vi "Overview.vi"() -> ()   [LabVIEW 2017]
panel:
  out "CTAH Temp In Res":dbl(graph)
  out "Heater Temp Out Res":dbl(graph)
  out "TCHX Temp In Res":dbl(graph)
  out "DHX Temp Out Res":dbl(graph)
  out "CTAH Heat Removal Res":dbl(graph)
  out "Heater Control Res":dbl(graph)
  out "Natural Gas Flow [kg/s]":sgl caption="C" format="%_3f"
  out "Time [s]":sgl format="%.1f"
  out "Primary Flow [kg/s]":sgl caption="C" format="%_3f"
  out "TCHX Power [W]":sgl caption="C" format="%_3f"
  out "DHX Power [W]":sgl caption="C" format="%_3f"
  out "Electrical Power [W]":sgl format="%_3f"
  in  "stop":bool
  out "Primary Min Temp [C]":sgl format="%_3f"
  out "CTAH Power [W]":sgl format="%_3f"
  out "Primary Max Temp [C]":sgl format="%_3f"
  out "Heater Power [W]":sgl caption="C" format="%_3f"
  out "LPT Work [W]":sgl format="%_3f"
  out "HPT Work [W]":sgl format="%_3f"
  out "Compressor Work [W]":sgl format="%_3f"
  out "Ambient Temperature [C]":sgl format="%_3f"
  # "Overview"
  # "TCHX"
  # "LPT"
  # "HPT"
  # "COMPRESSOR"
  # "DHX"
  # "CTAH"
  # "COMBUSTOR"
  # "HEATER"
  # "PUMP"
  # "NOAH Jr."
  # "Procedures"
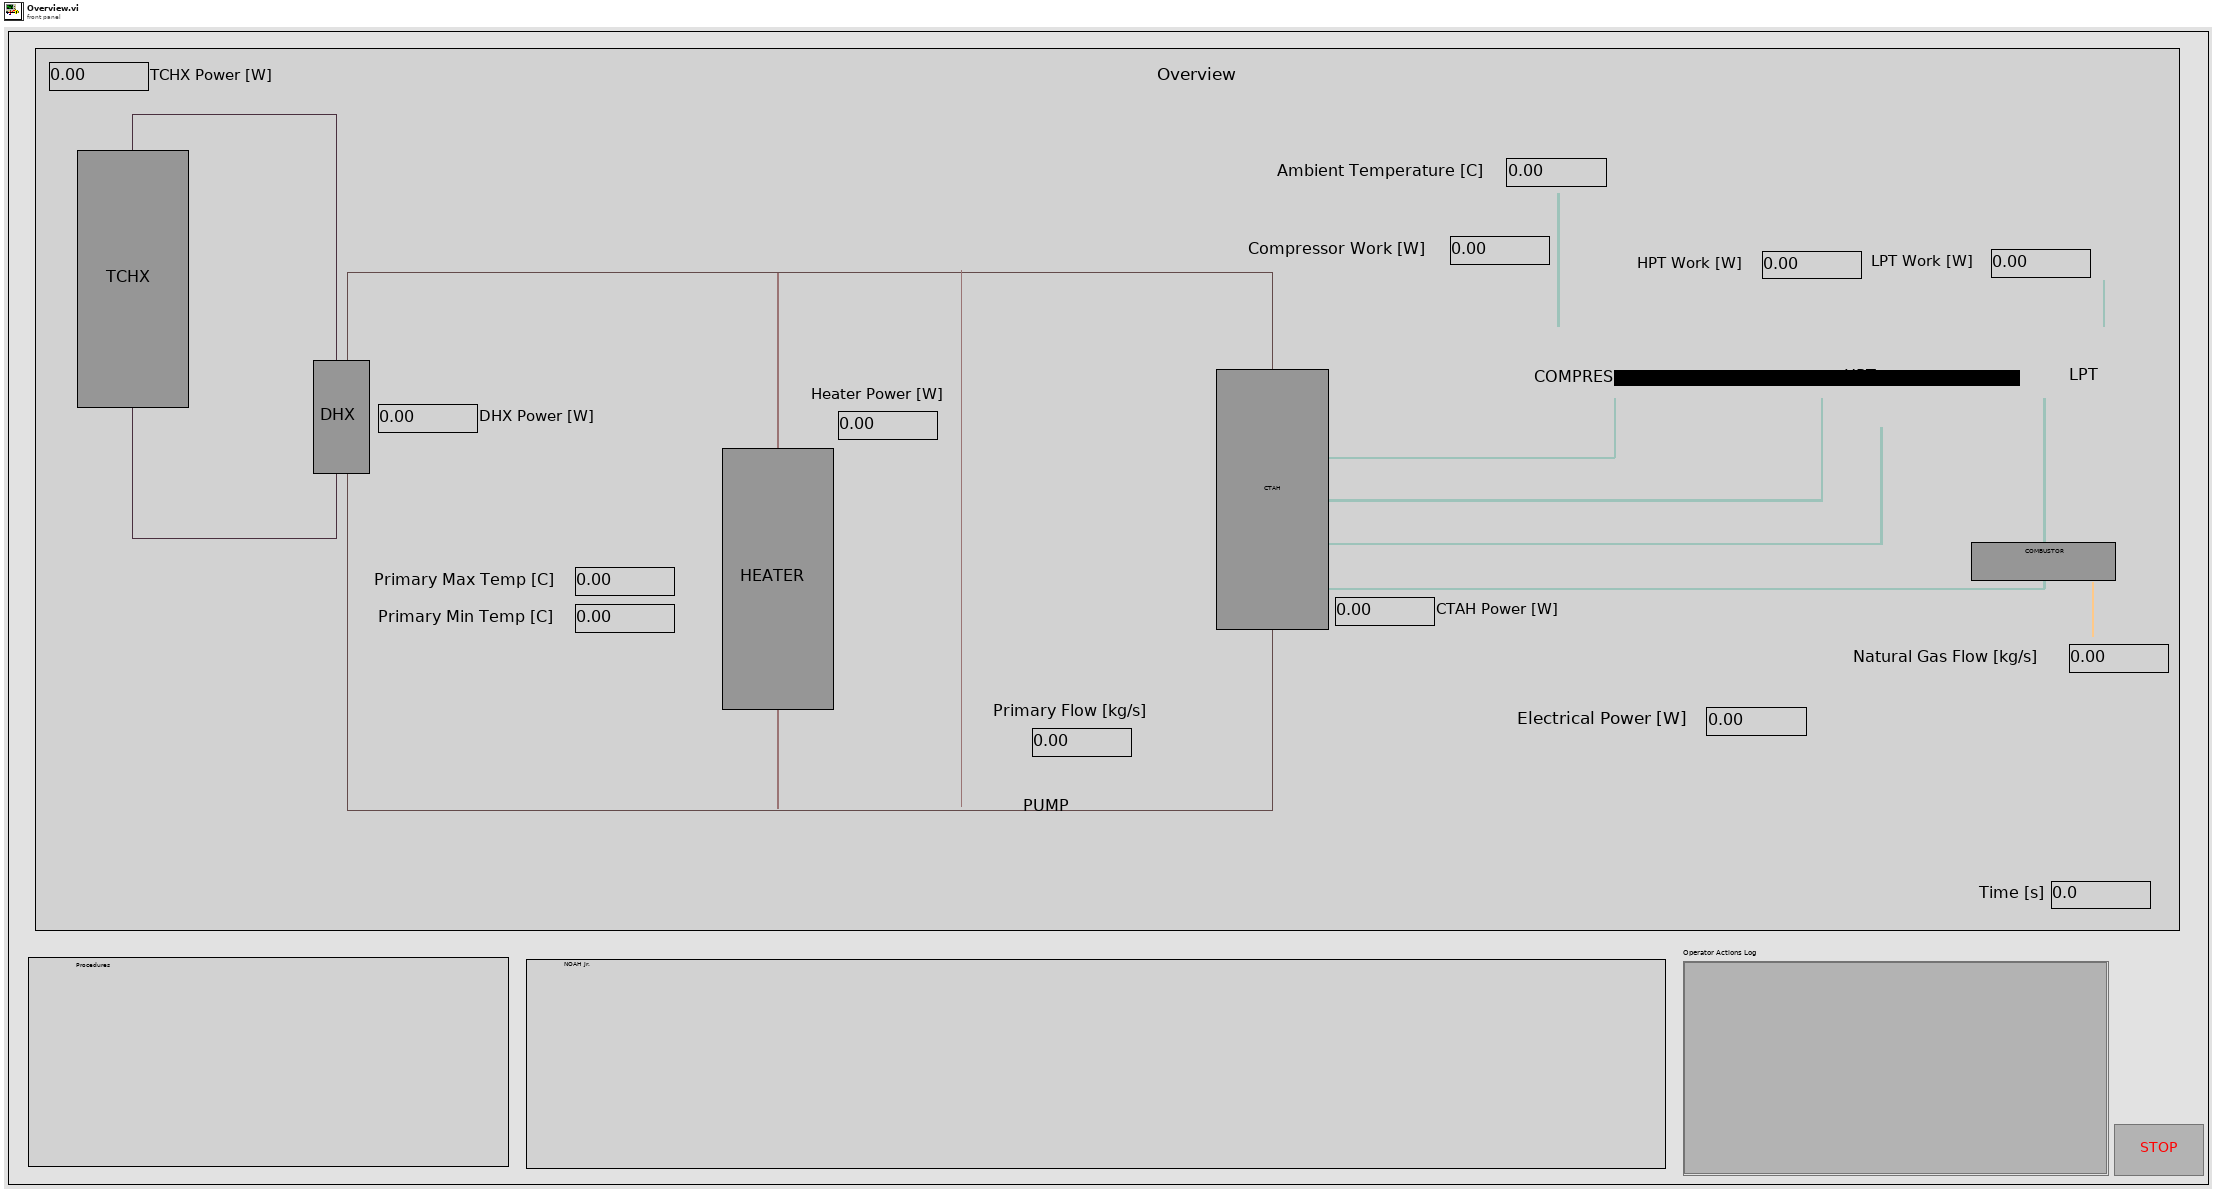
[diagram p1: front panel]
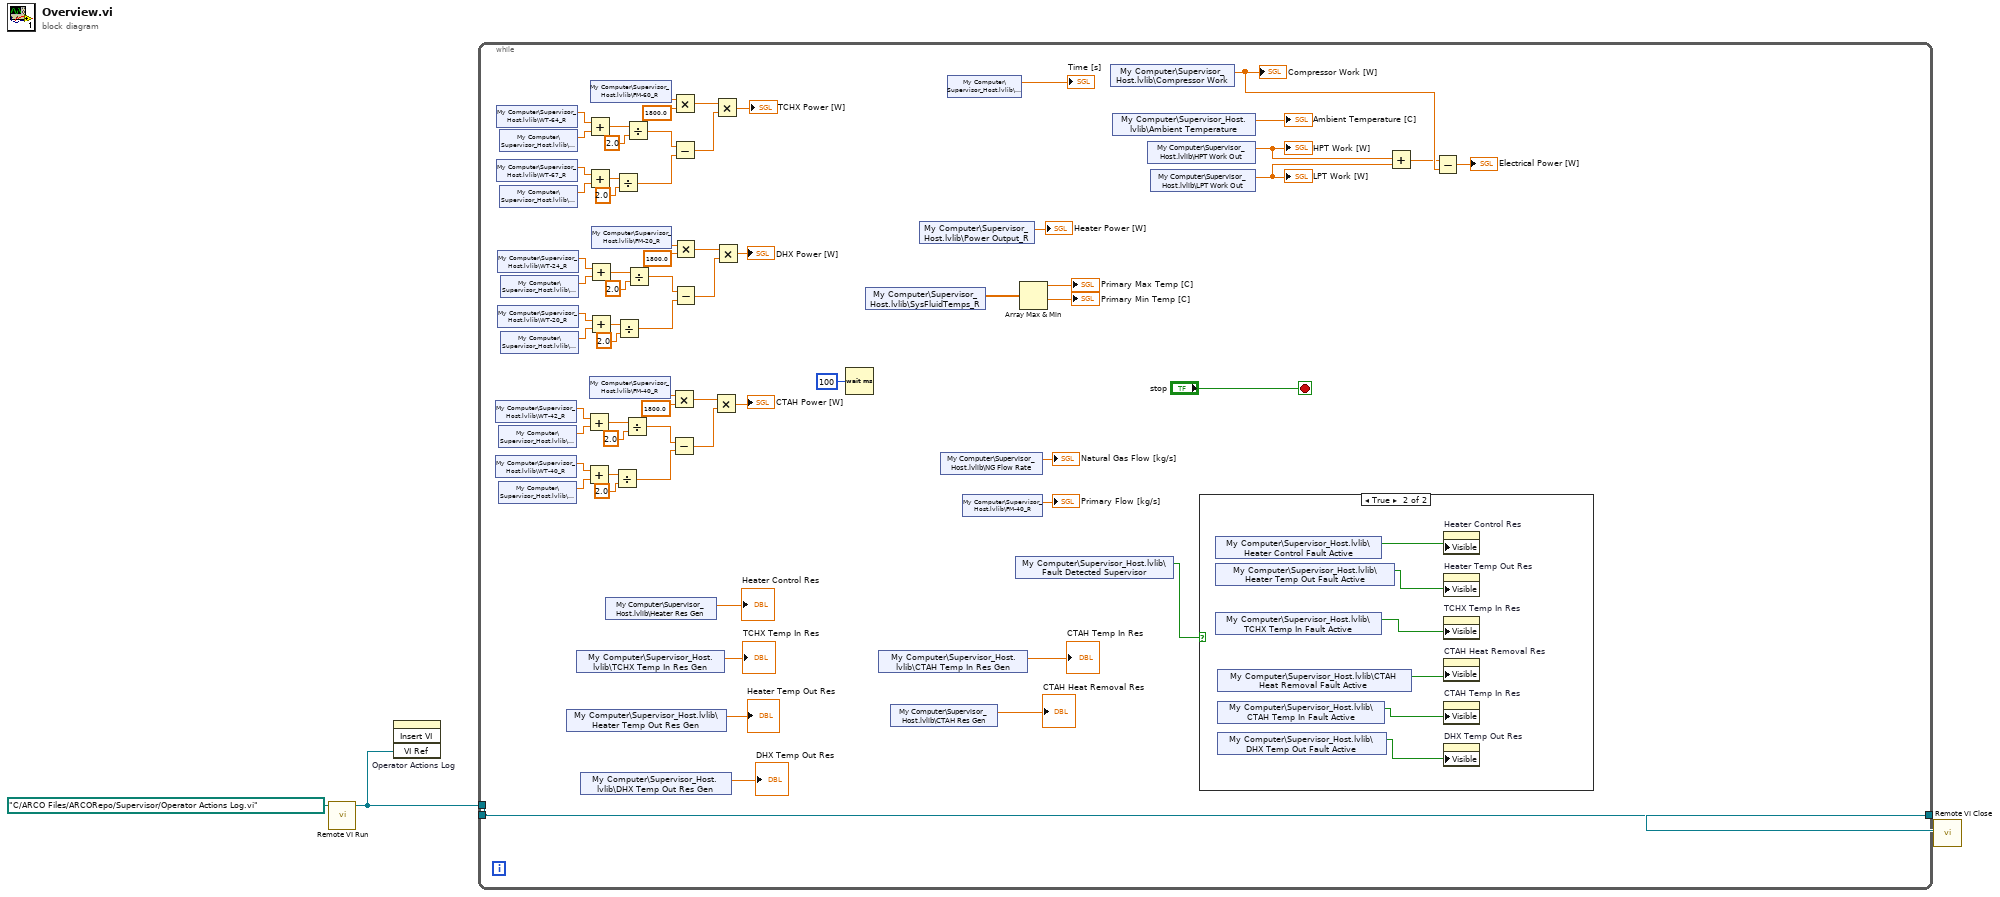
[diagram p0: block diagram]
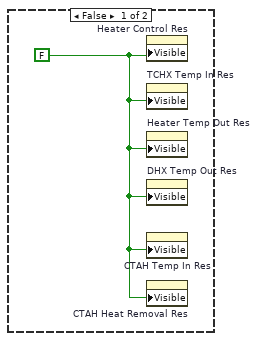
[diagram p2: hidden frame]
diagram:
  n1 = call "Remote VI Run.vi"("VI Path"=path "C:/ARCO Files/ARCORepo/Supervisor/Operator Actions Log.vi") -> ("VI Reference"=w2:refnum<vi>)  [unwired: 9 in, 1 out]
  n2 = invoke on="Operator Actions Log" class="SubPnl" method="Insert VI"("VI Ref"=w2) -> ()  [unwired: 3 in, 4 out]
  n3 = while {
    tunnel: [w5] -> _
    tunnel: w2 -> [w5]
    tunnel: [w5] -> w1
    stop <- "stop" stop-if-true
    n4 = shared-variable "My Computer\\Supervisor_Host.lvlib\\WT-42_R"() -> (w26:sgl)  [unwired: 1 in, 1 out]
    n5 = shared-variable "My Computer\\Supervisor_Host.lvlib\\WT-40_R"() -> (w23:sgl)  [unwired: 1 in, 1 out]
    n6 = shared-variable "My Computer\\Supervisor_Host.lvlib\\WT-64_R"() -> (w54:sgl)  [unwired: 1 in, 1 out]
    n7 = shared-variable "My Computer\\Supervisor_Host.lvlib\\WT-67_R"() -> (w51:sgl)  [unwired: 1 in, 1 out]
    n8 = shared-variable "My Computer\\Supervisor_Host.lvlib\\WT-24_R"() -> (w40:sgl)  [unwired: 1 in, 1 out]
    n9 = shared-variable "My Computer\\Supervisor_Host.lvlib\\WT-20_R"() -> (w37:sgl)  [unwired: 1 in, 1 out]
    n10 = shared-variable "My Computer\\Supervisor_Host.lvlib\\BT-43_R"() -> (w27:sgl)  [unwired: 1 in, 1 out]
    n11 = shared-variable "My Computer\\Supervisor_Host.lvlib\\BT-41_R"() -> (w22:sgl)  [unwired: 1 in, 1 out]
    n12 = shared-variable "My Computer\\Supervisor_Host.lvlib\\BT-65_R"() -> (w55:sgl)  [unwired: 1 in, 1 out]
    n13 = shared-variable "My Computer\\Supervisor_Host.lvlib\\BT-66_R"() -> (w50:sgl)  [unwired: 1 in, 1 out]
    n14 = shared-variable "My Computer\\Supervisor_Host.lvlib\\BT-25_R"() -> (w41:sgl)  [unwired: 1 in, 1 out]
    n15 = shared-variable "My Computer\\Supervisor_Host.lvlib\\BT-21_R"() -> (w36:sgl)  [unwired: 1 in, 1 out]
    n16 = shared-variable "My Computer\\Supervisor_Host.lvlib\\Heater Temp Out Res Gen"() -> (→"Heater Temp Out Res":dbl)  [unwired: 1 in, 1 out]
    n17 = shared-variable "My Computer\\Supervisor_Host.lvlib\\TCHX Temp In Res Gen"() -> (→"TCHX Temp In Res":dbl)  [unwired: 1 in, 1 out]
    n18 = shared-variable "My Computer\\Supervisor_Host.lvlib\\DHX Temp Out Res Gen"() -> (→"DHX Temp Out Res":dbl)  [unwired: 1 in, 1 out]
    n19 = Add(x=w26, y=w27) -> (x+y=w25:sgl)
    n20 = Add(x=w23, y=w22) -> (x+y=w21:sgl)
    n21 = Add(x=w54, y=w55) -> (x+y=w53:sgl)
    n22 = Add(x=w51, y=w50) -> (x+y=w49:sgl)
    n23 = Add(x=w40, y=w41) -> (x+y=w39:sgl)
    n24 = Add(x=w37, y=w36) -> (x+y=w35:sgl)
    n25 = shared-variable "My Computer\\Supervisor_Host.lvlib\\FM-40_R"() -> (w29:sgl)  [unwired: 1 in, 1 out]
    n26 = shared-variable "My Computer\\Supervisor_Host.lvlib\\FM-60_R"() -> (w57:sgl)  [unwired: 1 in, 1 out]
    n27 = shared-variable "My Computer\\Supervisor_Host.lvlib\\FM-20_R"() -> (w43:sgl)  [unwired: 1 in, 1 out]
    n28 = shared-variable "My Computer\\Supervisor_Host.lvlib\\Heater Res Gen"() -> (→"Heater Control Res":dbl)  [unwired: 1 in, 1 out]
    n29 = Divide(x=w21, y=sgl 2.0) -> (x/y=w18:sgl)
    n30 = Divide(x=w49, y=sgl 2.0) -> (x/y=w46:sgl)
    n31 = Divide(x=w35, y=sgl 2.0) -> (x/y=w32:sgl)
    n32 = Divide(x=w25, y=sgl 2.0) -> (x/y=w19:sgl)
    n33 = Divide(x=w53, y=sgl 2.0) -> (x/y=w47:sgl)
    n34 = Divide(x=w39, y=sgl 2.0) -> (x/y=w33:sgl)
    n35 = Multiply(x=w29, y=sgl 1800.0) -> (x*y=w17:sgl)
    n36 = Subtract(x=w19, y=w18) -> (x-y=w16:sgl)
    n37 = Multiply(x=w57, y=sgl 1800.0) -> (x*y=w45:sgl)
    n38 = Subtract(x=w47, y=w46) -> (x-y=w44:sgl)
    n39 = Multiply(x=w43, y=sgl 1800.0) -> (x*y=w31:sgl)
    n40 = Subtract(x=w33, y=w32) -> (x-y=w30:sgl)
    n41 = Multiply(x=w17, y=w16) -> (x*y=→"CTAH Power [W]":sgl)
    n42 = Multiply(x=w45, y=w44) -> (x*y=→"TCHX Power [W]":sgl)
    n43 = Multiply(x=w31, y=w30) -> (x*y=→"DHX Power [W]":sgl)
    n44 = Wait (ms)(milliseconds to wait=u32 100) -> ()  [unwired: 1 out]
    n45 = shared-variable "My Computer\\Supervisor_Host.lvlib\\SysFluidTemps_R"() -> (w70:sgl[])  [unwired: 1 in, 1 out]
    n46 = shared-variable "My Computer\\Supervisor_Host.lvlib\\CTAH Temp In Res Gen"() -> (→"CTAH Temp In Res":dbl)  [unwired: 1 in, 1 out]
    n47 = shared-variable "My Computer\\Supervisor_Host.lvlib\\CTAH Res Gen"() -> (→"CTAH Heat Removal Res":dbl)  [unwired: 1 in, 1 out]
    n48 = shared-variable "My Computer\\Supervisor_Host.lvlib\\Power Output_R"() -> (→"Heater Power [W]":sgl)  [unwired: 1 in, 1 out]
    n49 = shared-variable "My Computer\\Supervisor_Host.lvlib\\NG Flow Rate"() -> (→"Natural Gas Flow [kg/s]":sgl)  [unwired: 1 in, 1 out]
    n50 = shared-variable "My Computer\\Supervisor_Host.lvlib\\Time_R"() -> (→"Time [s]":sgl)  [unwired: 1 in, 1 out]
    n51 = shared-variable "My Computer\\Supervisor_Host.lvlib\\FM-40_R"() -> (→"Primary Flow [kg/s]":sgl)  [unwired: 1 in, 1 out]
    n52 = shared-variable "My Computer\\Supervisor_Host.lvlib\\Fault Detected Supervisor"() -> (w4:bool)  [unwired: 1 in, 1 out]
    n53 = Array Max & Min(array=w70) -> (max value=→"Primary Max Temp [C]":sgl, min value=→"Primary Min Temp [C]":sgl)  [unwired: 2 out]
    n54 = shared-variable "My Computer\\Supervisor_Host.lvlib\\Compressor Work"() -> (w61:sgl)  [unwired: 1 in, 1 out]
    "Compressor Work [W]" <- w61
    n55 = shared-variable "My Computer\\Supervisor_Host.lvlib\\Ambient Temperature"() -> (→"Ambient Temperature [C]":sgl)  [unwired: 1 in, 1 out]
    n56 = shared-variable "My Computer\\Supervisor_Host.lvlib\\HPT Work Out"() -> (w63:sgl)  [unwired: 1 in, 1 out]
    "HPT Work [W]" <- w63
    n57 = shared-variable "My Computer\\Supervisor_Host.lvlib\\LPT Work Out"() -> (w62:sgl)  [unwired: 1 in, 1 out]
    "LPT Work [W]" <- w62
    n58 = case shown="True" w4 {
      frame False {
        w72 = FALSE
        n59 = property on="Heater Control Res" class="WFChart (strict)"("Visible"=w72) -> ()  [unwired: 2 in, 2 out]
        n60 = property on="TCHX Temp In Res" class="WFChart (strict)"("Visible"=w72) -> ()  [unwired: 2 in, 2 out]
        n61 = property on="Heater Temp Out Res" class="WFChart (strict)"("Visible"=w72) -> ()  [unwired: 2 in, 2 out]
        n62 = property on="DHX Temp Out Res" class="WFChart (strict)"("Visible"=w72) -> ()  [unwired: 2 in, 2 out]
        n63 = property on="CTAH Temp In Res" class="WFChart (strict)"("Visible"=w72) -> ()  [unwired: 2 in, 2 out]
        n64 = property on="CTAH Heat Removal Res" class="WFChart (strict)"("Visible"=w72) -> ()  [unwired: 2 in, 2 out]
      }
      frame True {
        n65 = shared-variable "My Computer\\Supervisor_Host.lvlib\\Heater Control Fault Active"() -> (w78:bool)  [unwired: 1 in, 1 out]
        n66 = shared-variable "My Computer\\Supervisor_Host.lvlib\\Heater Temp Out Fault Active"() -> (w77:bool)  [unwired: 1 in, 1 out]
        n67 = shared-variable "My Computer\\Supervisor_Host.lvlib\\TCHX Temp In Fault Active"() -> (w76:bool)  [unwired: 1 in, 1 out]
        n68 = shared-variable "My Computer\\Supervisor_Host.lvlib\\CTAH Heat Removal Fault Active"() -> (w75:bool)  [unwired: 1 in, 1 out]
        n69 = shared-variable "My Computer\\Supervisor_Host.lvlib\\CTAH Temp In Fault Active"() -> (w74:bool)  [unwired: 1 in, 1 out]
        n70 = shared-variable "My Computer\\Supervisor_Host.lvlib\\DHX Temp Out Fault Active"() -> (w73:bool)  [unwired: 1 in, 1 out]
        n71 = property on="Heater Control Res" class="WFChart (strict)"("Visible"=w78) -> ()  [unwired: 2 in, 2 out]
        n72 = property on="Heater Temp Out Res" class="WFChart (strict)"("Visible"=w77) -> ()  [unwired: 2 in, 2 out]
        n73 = property on="TCHX Temp In Res" class="WFChart (strict)"("Visible"=w76) -> ()  [unwired: 2 in, 2 out]
        n74 = property on="CTAH Heat Removal Res" class="WFChart (strict)"("Visible"=w75) -> ()  [unwired: 2 in, 2 out]
        n75 = property on="CTAH Temp In Res" class="WFChart (strict)"("Visible"=w74) -> ()  [unwired: 2 in, 2 out]
        n76 = property on="DHX Temp Out Res" class="WFChart (strict)"("Visible"=w73) -> ()  [unwired: 2 in, 2 out]
      }
    }
    n77 = Add(x=w63, y=w62) -> (x+y=w60:sgl)
    n78 = Subtract(x=w60, y=w61) -> (x-y=→"Electrical Power [W]":sgl)
  }
  n79 = call "Remote VI Close.vi"("reference"=w1) -> ()  [unwired: 9 in, 2 out]
